vi "Stepper.vi"() -> ()   [LabVIEW 2011]
uses:
  <vilib>/LabVIEW Interface for Arduino/Type Defs/Board Type.ctl
  <vilib>/LabVIEW Interface for Arduino/LabVIEW Interface for Arduino.lvlib
panel:
  out "Ready?":bool
  in  "stop":bool
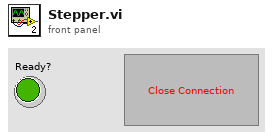
[diagram p1: front panel]
types:
  T1 = typedef "LabVIEW Interface for Arduino.lvlib/Board Type.ctl" = enum16{"Uno", "Dimuelanove w/Atmega 328", "Mega 2560"}
  T2 = typedef "LabVIEW Interface for Arduino.lvlib/Arduino Resource.ctl" = cluster{"VISA resource":refnum<visa-resource-name>, "Board Type":T1, "Connection Type":enum8{"USB / Serial"}, "Bytes Per Packet (15)":u8}
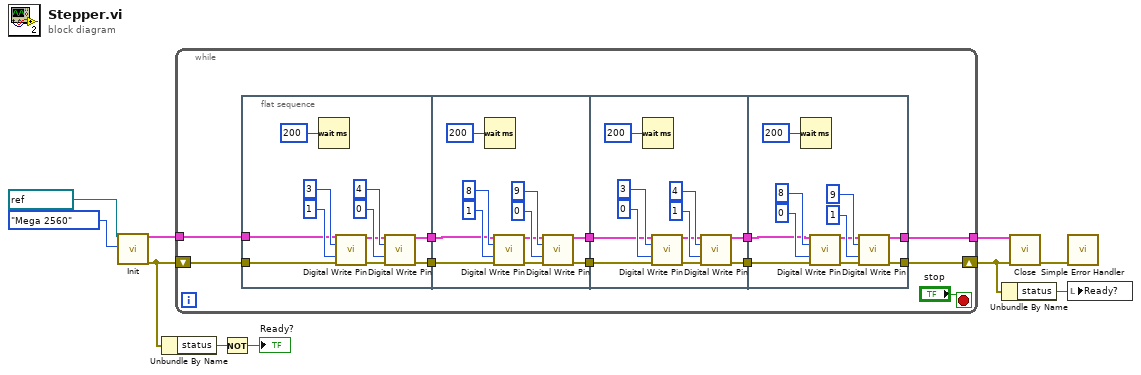
[diagram p0: block diagram]
diagram:
  n1 = call <vilib>:"Init.vi"("VISA resource"=refnum<visa-resource-name> "COM3", "Board Type (Uno)"=Board_Type."Mega 2560") -> ("Arduino Resource"=w5:T2, "error out"=w4:errorcluster)  [unwired: 16 in]
  n2 = Unbundle By Name(w4) -> ("status"=w7:bool)
  n3 = while {
    tunnel: w5 -> [w14]
    shift-right: [w12] -> w2
    shift-left: w4 -> [w13]
    tunnel: [w11] -> w3
    stop <- "stop" stop-if-true
    n4 = flat-sequence {
      tunnel: [w25] -> w20
      tunnel: [w24] -> w19
      tunnel: w14 -> [w23]
      tunnel: w13 -> [w22]
      tunnel: w20 -> [w36]
      tunnel: [w35] -> w18
      tunnel: w19 -> [w34]
      tunnel: [w33] -> w17
      tunnel: w18 -> [w47]
      tunnel: [w46] -> w16
      tunnel: w17 -> [w45]
      tunnel: [w44] -> w15
      tunnel: w16 -> [w58]
      tunnel: w15 -> [w57]
      tunnel: [w56] -> w12
      tunnel: [w55] -> w11
      frame #0 {
        n5 = Wait (ms)(milliseconds to wait=u32 200) -> ()  [unwired: 1 out]
        n6 = call <vilib>:"Digital Write Pin.vi"("Arduino Resource"=w23, "Digital I/O Pin (0)"=u8 3, "Value (0)"=u8 1, "error in"=w22) -> ("Arduino Resource"=w29:T2, "error out"=w28:errorcluster)  [unwired: 10 in]
        n7 = call <vilib>:"Digital Write Pin.vi"("Arduino Resource"=w29, "Digital I/O Pin (0)"=u8 4, "Value (0)"=u8 0, "error in"=w28) -> ("Arduino Resource"=w25:T2, "error out"=w24:errorcluster)  [unwired: 10 in]
      }
      frame #1 {
        n8 = Wait (ms)(milliseconds to wait=u32 200) -> ()  [unwired: 1 out]
        n9 = call <vilib>:"Digital Write Pin.vi"("Arduino Resource"=w36, "Digital I/O Pin (0)"=u8 8, "Value (0)"=u8 1, "error in"=w34) -> ("Arduino Resource"=w40:T2, "error out"=w39:errorcluster)  [unwired: 10 in]
        n10 = call <vilib>:"Digital Write Pin.vi"("Arduino Resource"=w40, "Digital I/O Pin (0)"=u8 9, "Value (0)"=u8 0, "error in"=w39) -> ("Arduino Resource"=w35:T2, "error out"=w33:errorcluster)  [unwired: 10 in]
      }
      frame #2 {
        n11 = Wait (ms)(milliseconds to wait=u32 200) -> ()  [unwired: 1 out]
        n12 = call <vilib>:"Digital Write Pin.vi"("Arduino Resource"=w47, "Digital I/O Pin (0)"=u8 3, "Value (0)"=u8 0, "error in"=w45) -> ("Arduino Resource"=w51:T2, "error out"=w50:errorcluster)  [unwired: 10 in]
        n13 = call <vilib>:"Digital Write Pin.vi"("Arduino Resource"=w51, "Digital I/O Pin (0)"=u8 4, "Value (0)"=u8 1, "error in"=w50) -> ("Arduino Resource"=w46:T2, "error out"=w44:errorcluster)  [unwired: 10 in]
      }
      frame #3 {
        n14 = Wait (ms)(milliseconds to wait=u32 200) -> ()  [unwired: 1 out]
        n15 = call <vilib>:"Digital Write Pin.vi"("Arduino Resource"=w58, "Digital I/O Pin (0)"=u8 8, "Value (0)"=u8 0, "error in"=w57) -> ("Arduino Resource"=w62:T2, "error out"=w61:errorcluster)  [unwired: 10 in]
        n16 = call <vilib>:"Digital Write Pin.vi"("Arduino Resource"=w62, "Digital I/O Pin (0)"=u8 9, "Value (0)"=u8 1, "error in"=w61) -> ("Arduino Resource"=w55:T2, "error out"=w56:errorcluster)  [unwired: 10 in]
      }
    }
  }
  n17 = Not(x=w7) -> (.not. x?=→"Ready?":bool)
  n18 = Unbundle By Name(w2) -> ("status"=w1:bool)
  n19 = call <vilib>:"Close.vi"("Arduino Resource"=w3, "error in"=w2) -> ("error out"=w9:errorcluster)  [unwired: 13 in]
  n20 = call <vilib>:"Simple Error Handler.vi"("error in (no error)"=w9) -> ()  [unwired: 4 in, 5 out]
  n21 = local write "Ready?"(w1) -> ()
